vi "util.fixViPanes.vi"(11 "VI in":refnum<vi>) -> ()   [LabVIEW 2024]
uses:
  <vilib>/Utility/miscctls.llb/LVPointTypeDef.ctl
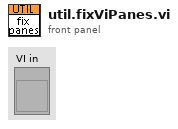
[diagram p1: front panel]
types:
  T1 = typedef "LVPointTypeDef.ctl" = cluster{"Horizontal":i16, "Vertical":i16}
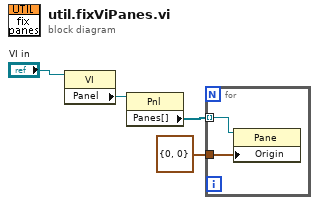
[diagram p0: block diagram]
diagram:
  n1 = property class="VI"(reference="VI in") -> ("Panel"=w1:refnum<vi>)  [unwired: 1 in, 2 out]
  n2 = property class="Pnl"(reference=w1) -> ("Panes[]"=w3:refnum<vi>[])  [unwired: 1 in, 2 out]
  n3 = for {
    tunnel: w3 -> [w6] mode=indexing
    tunnel: T1 {"Horizontal"=0, "Vertical"=0} ("Origin") -> [w5]
    n4 = property class="Pane"(reference=w6, "Origin"=w5) -> ()  [unwired: 1 in, 2 out]
  }
